vi "Launch Connection Handler.vi"(6 "timeout ms (5000)":i32=5000, 7 "Connection Handler Reference":refnum<vi>, 8 "error in (no error)":errorcluster, 9 "Remote Address":string, 10 "WebSocket Connection in":refnum<k5>, 11 "References In":variant) -> (0 "error out":errorcluster)   [LabVIEW 2013, in "WebSocket Server.lvlib"]
uses:
  WebSocket Server.lvlib
  <vilib>/Intelligent Energy/WebSockets API/WebSockets/WebSockets.lvlib
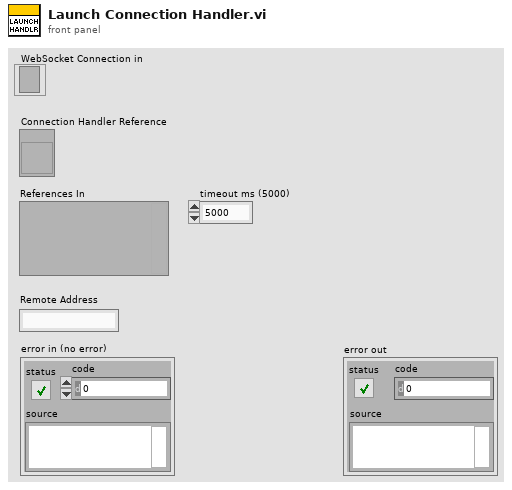
[diagram p1: front panel]
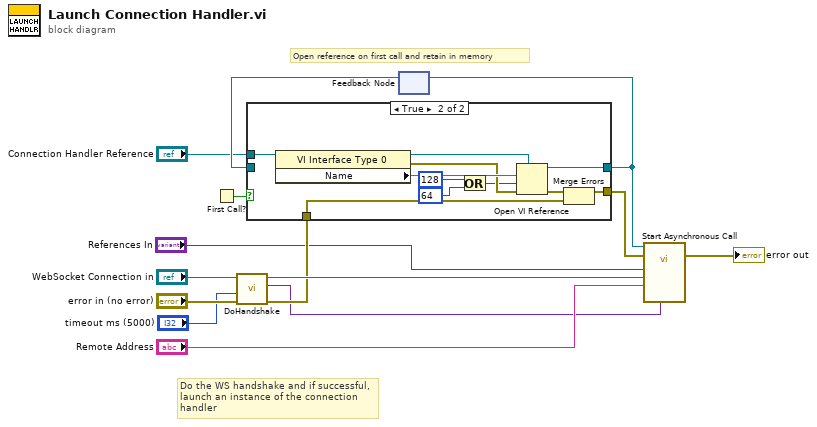
[diagram p0: block diagram]
diagram:
  # "Open reference on first call and retain in memory"
  # "Do the WS handshake and if successful, launch an instance of the connection handler"
  n1 = First Call?() -> (First Call?: T/F=w6:bool)
  n2 = call <vilib>:"DoHandshake.vi"("error in (no error)"="error in (no error)", "timeout ms (5000)"="timeout ms (5000)", "WebSocket Connection in"="WebSocket Connection in") -> ("error out"=w11:errorcluster, "Headers Out"=w7:variant, "WebSocket Connection out"=w13:refnum<k5>)  [unwired: 5 in, 1 out]
  n3 = feedback #1() -> (w4:refnum<vi>)  [unwired: 1 in]
  n4 = case shown="True" w6 {
    tunnel: [w16 w24] -> w5
    tunnel: [w15 w22] -> w12
    tunnel: w11 -> [w15 w21]
    tunnel: w4 -> [w16 _]
    tunnel: "Connection Handler Reference" -> [_ w20]
    frame False {
    }
    frame True {
      n5 = property class="VI Interface Type 0"(reference=w20) -> (reference out=w27:refnum<vi>, error out=w25:errorcluster, "Name"=w26:string)  [unwired: 1 in]
      n6 = Or(x=128 ("options"), y=64 ("options")) -> (x .or. y?=w19:i32)
      n7 = Open VI Reference(type specifier VI Refnum (for type only)=w27, vi path=w26, options=w19, error in (no error)=w25) -> (vi reference=w24:refnum<vi>, error out=w23:errorcluster)  [unwired: 2 in]
      n8 = Merge Errors(w23, w21) -> (w22:errorcluster)
    }
  }
  n9 = feedback-in #1(w5) -> ()
  n10 = call-by-ref "Start Asynchronous Call"(reference=w5, error in=w12, "WebSocket Headers"=w7, "Remote Address"="Remote Address", "connection ID"=w13, "References In"="References In") -> (error out=→"error out":errorcluster)  [unwired: 7 in, 2 out]
